vi "ParseRulesFile.vi"(8 "error in (no error)":errorcluster, 9 "Parameters":string, 11 "CDefaultRuleFileParser in":refnum<class "CDefaultRuleFileParser.lvclass">) -> (0 "error out":errorcluster, 2 "Rules":T1, 3 "CDefaultRuleFileParser out":refnum<class "CDefaultRuleFileParser.lvclass">)   [LabVIEW 2020, in "DefaultExtensions.lvlib" / "CDefaultRuleFileParser.lvclass"]
uses:
  CDefaultRuleFileParser.lvclass
  ExtensionInterfaces/IRuleFileParser/RulesDefinition.ctl
  Private/Paramters.ctl
  <vilib>/xml/Load XML File.vi
  <vilib>/xml/Close Reference(Node).vi
  <vilib>/xml/NI_XML.lvlib
  ExtensionInterfaces/IRuleFileParser/IRuleFileParser.lvclass
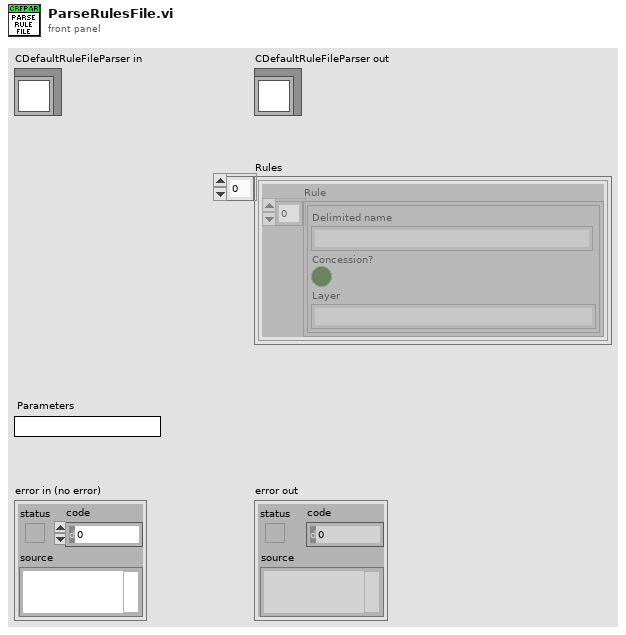
[diagram p1: front panel]
types:
  T1 = typedef "ExtensionInterfaces.lvlib/IRuleFileParser.lvclass/RulesDefinition.ctl" = cluster{"Rule":cluster{"Delimited name":string, "Concession?":bool, "Layer":string}[]}[]
  T2 = typedef "DefaultExtensions.lvlib/CDefaultRuleFileParser.lvclass/Paramters.ctl" = cluster{"Path":string}
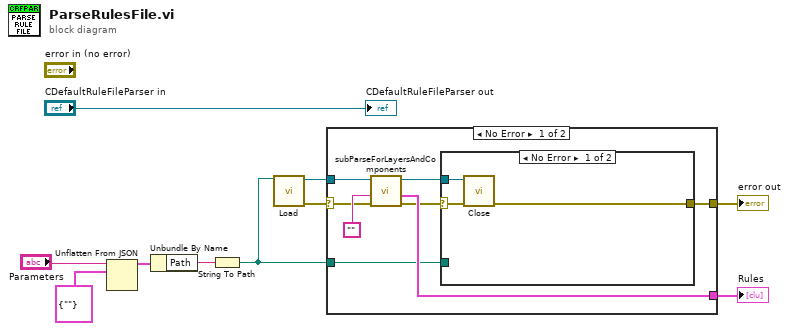
[diagram p0: block diagram]
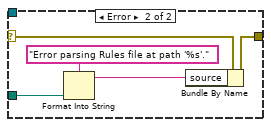
[diagram p2: hidden frame]
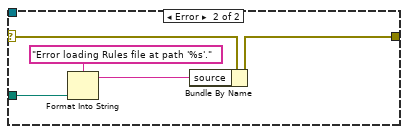
[diagram p3: hidden frame]
diagram:
  n1 = Unflatten From JSON(JSON string="Parameters", type and defaults=T2 {"Path"=""} ("Parameters")) -> (value=w4:T2)  [unwired: 5 in, 1 out]
  n2 = Unbundle By Name(w4) -> ("Path"=w3:string)
  n3 = String To Path(string=w3) -> (path=w2:path)
  n4 = call-poly <vilib>:"Load.vi"("path to XML document"=w2) -> ("DOM document out"=w9:refnum<k20>, "error out"=w7:errorcluster)  [unwired: 12 in, 1 out]
  n5 = case shown="No Error" w7 {
    selector: w7 -> [w14 w29]
    tunnel: w9 -> [w16 _]
    tunnel: [w15 _] -> w8
    tunnel: [w12 w28] -> w6
    tunnel: w2 -> [w11 w27]
    frame No Error {
      n6 = call "subParseForLayersAndComponents.vi"("error in (no error)"=w14, "Parent node"="", "Refnum in"=w16) -> ("error out"=w13:errorcluster, "Rules"=w15:T1, "Refnum out"=w18:refnum<k20>)  [unwired: 6 in]
      n7 = case shown="No Error" w13 {
        selector: w13 -> [w20 w24]
        tunnel: w18 -> [w21 _]
        tunnel: [w19 w23] -> w12
        tunnel: w11 -> [_ w22]
        frame No Error {
          n8 = call-poly <vilib>:"Close.vi"("error in (no error)"=w20, "node"=w21) -> ("error out"=w19:errorcluster)  [unwired: 7 in]
        }
        frame Error {
          n9 = Format Into String(format string="Error parsing Rules file at path '%s'.", w22) -> (resulting string=w26:string)  [unwired: 2 in, 1 out]
          n10 = Bundle By Name(cluster=w24, "source"=w26) -> (w23:errorcluster)
        }
      }
    }
    frame Error {
      n11 = Format Into String(format string="Error loading Rules file at path '%s'.", w27) -> (resulting string=w31:string)  [unwired: 2 in, 1 out]
      n12 = Bundle By Name(cluster=w29, "source"=w31) -> (w28:errorcluster)
    }
  }
  "error out" <- w6
  "Rules" <- w8
  "CDefaultRuleFileParser out" <- "CDefaultRuleFileParser in"
